vi "User@TabTrigger__Parameter.vi"(1 "ParamterIn":string) -> (0 "ParamterOut":string)   [LabVIEW 2020]
panel:
  in  "Parameters":string(combo)
  in  "UserPanelControl":string(combo)
  in  "Confirm":bool
  # "User@TabTrigger $UserPanelControlName,$TabIndex"
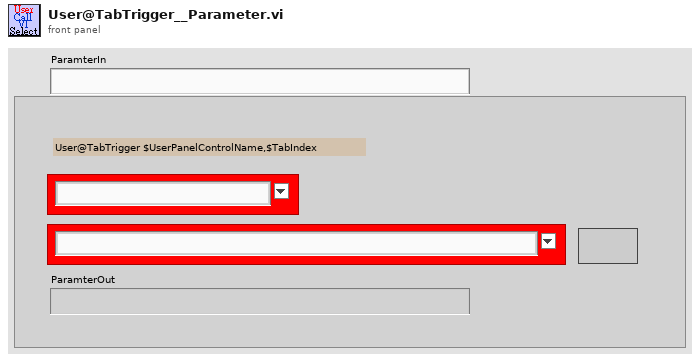
[diagram p1: front panel]
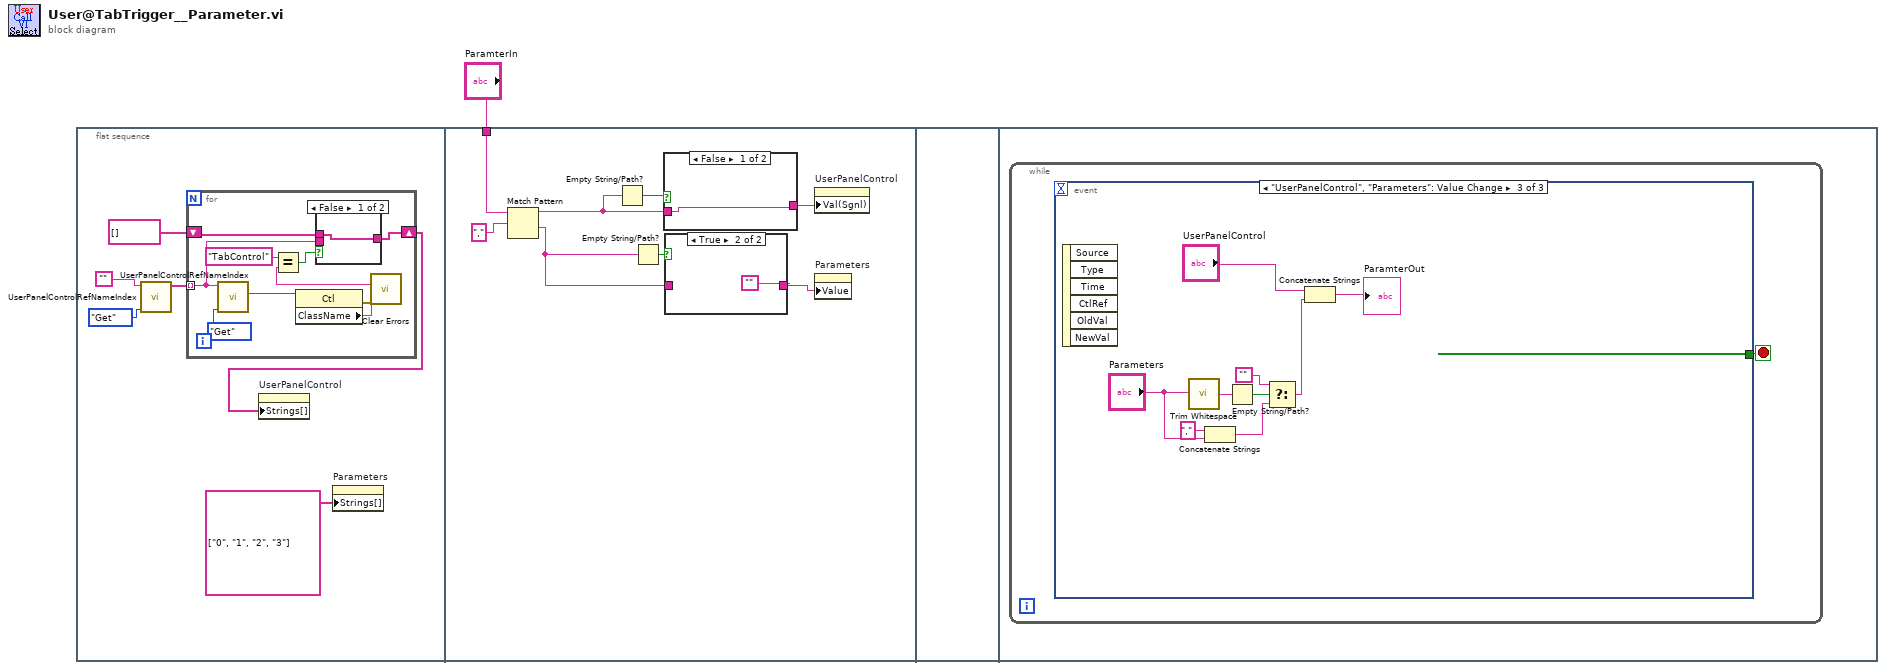
[diagram p0: block diagram]
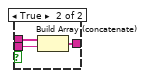
[diagram p2: hidden frame]
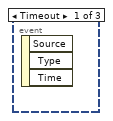
[diagram p5: hidden frame]
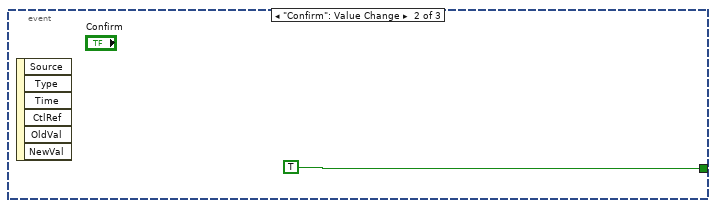
[diagram p6: hidden frame]
diagram:
  n1 = flat-sequence {
    tunnel: "ParamterIn" -> [w26]
    frame #0 {
      n2 = call "UserPanelControlRefNameIndex.vi"("OP"=enum16{"Get", "Update", "Init"}."Get", "ControlName"="") -> ("ControlNameS"=w5:string[])  [unwired: 6 in, 3 out]
      n3 = for {
        tunnel: w5 -> [w11] mode=indexing
        shift-right: [w10] -> w3
        shift-left: string[] [] ("Strings []") -> [w12]
        n4 = call "UserPanelControlRefNameIndex.vi"("OP"=enum16{"Get", "Update", "Init"}."Get", "ControlName"=w11) -> ("ControlRefOut"=w15:refnum<vi>)  [unwired: 6 in, 3 out]
        n5 = property class="Ctl"(reference=w15) -> (error out=w8:errorcluster, "ClassName"=w14:string)  [unwired: 1 in, 1 out]
        n6 = Equal?(x="TabControl" ("Class Name"), y=w14) -> (x = y?=w13:bool)
        n7 = case shown="False" w13 {
          tunnel: w12 -> [w17 w20]
          tunnel: w11 -> [_ w19]
          tunnel: [w17 w18] -> w10
          frame False {
          }
          frame True {
            n8 = Build Array (concatenate)(w20, w19) -> (w18:string[])
          }
        }
        n9 = call <vilib>:"Clear Errors.vi"("error in (no error)"=w8) -> ()  [unwired: 5 in, 2 out]
      }
      n10 = property on="UserPanelControl" class="CmbBox"("Strings[]"=w3) -> ()  [unwired: 2 in, 2 out]
      n11 = property on="Parameters" class="CmbBox"("Strings[]"=string[] ["0", "1", "2", "3"] ("Strings []")) -> ()  [unwired: 2 in, 2 out]
    }
    frame #1 {
      n12 = Match Pattern(string=w26, regular expression=",") -> (before substring=w24:string, after substring=w23:string)  [unwired: 1 in, 2 out]
      n13 = Empty String/Path?(string/path=w24) -> (empty?=w28:bool)
      n14 = Empty String/Path?(string/path=w23) -> (empty?=w27:bool)
      n15 = case shown="False" w28 {
        tunnel: w24 -> [w31 w32]
        tunnel: [w31 w32] -> w21
        frame False {
        }
        frame True {
        }
      }
      n16 = case shown="True" w27 {
        tunnel: [w29 ""] -> w22
        tunnel: w23 -> [w29 _]
        frame False {
        }
        frame True {
        }
      }
      n17 = property on="UserPanelControl" class="CmbBox"("Val(Sgnl)"=w21) -> ()  [unwired: 2 in, 2 out]
      n18 = property on="Parameters" class="CmbBox"("Value"=w22) -> ()  [unwired: 2 in, 2 out]
    }
    frame #2 {
    }
    frame #3 {
      n19 = while {
        stop <- w33 stop-if-true
        n20 = event shown="[2] \"UserPanelControl\", \"Parameters\": Value Change" {
          selector: _ -> [_ _ _]
          dyn-events: _ -> [_ _ _]
          timeout: _ -> [_ _ _]
          tunnel: [_ TRUE _] -> w33
          event Timeout {
            n21 = event-data() -> ()  [unwired: 1 in, 3 out]
          }
          event "Confirm": Value Change {
            n22 = event-data() -> ()  [unwired: 1 in, 6 out]
          }
          event "UserPanelControl", "Parameters": Value Change {
            n23 = event-data() -> ()  [unwired: 1 in, 6 out]
            n24 = call <vilib>:"Trim Whitespace.vi"("string"="Parameters") -> ("trimmed string"=w39:string)  [unwired: 1 in]
            n25 = Concatenate Strings("," ("string"), "Parameters") -> (w38:string)
            n26 = Empty String/Path?(string/path=w39) -> (empty?=w40:bool)
            n27 = Select(t="", s=w40, f=w38) -> (s? t:f=w35:string)
            n28 = Concatenate Strings("UserPanelControl", w35) -> (→"ParamterOut":string)
          }
        }
      }
    }
  }
